vi "RegisterMap_Split RegMap.vi"(8 "error in (no error)":errorcluster, 11 "Register RegMap Strings":string[](array[string])) -> (0 "error out":errorcluster, 2 "Register RegMap Data":string[][](array[string]))   [LabVIEW 2010]
doc: "This VI splits the RegMap string from the text file into the individual bits/components.\n\nInputs:\nRegister RegMap Strings - (str[]) array of strings containing the specific register format for each of the regsiters in the register map file; rows = register and its format\nerror in - error input cluster\n\nOutputs:\nRegister RegMap Data - (str[]) 2-D array of strings with a element in the array for each register's format\nerror out - error output cluster"
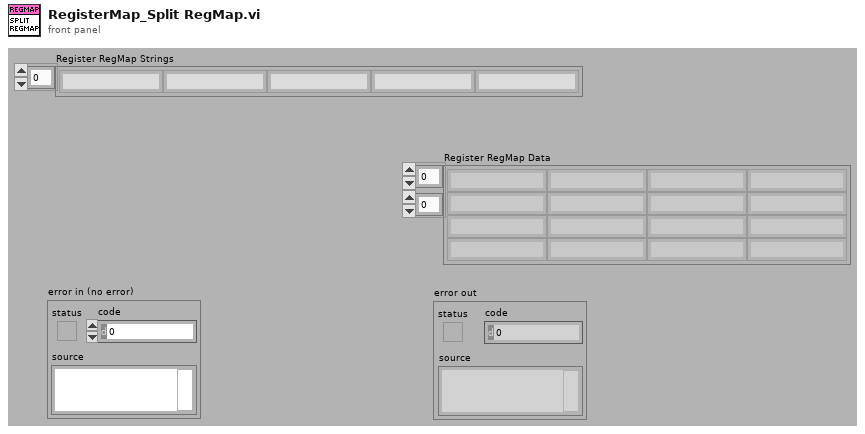
[diagram p1: front panel]
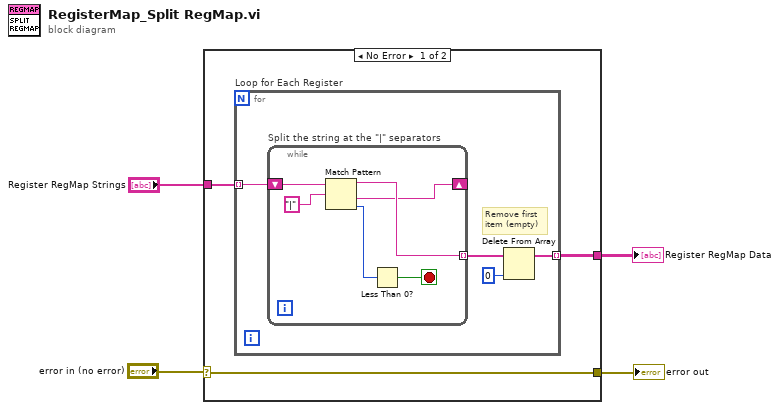
[diagram p0: block diagram]
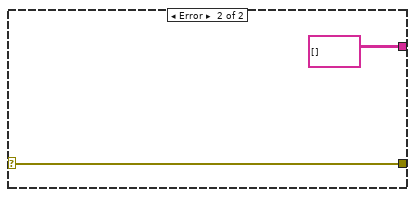
[diagram p2: hidden frame]
diagram:
  n1 = case shown="No Error" "error in (no error)" {
    selector: "error in (no error)" -> [w5 w19]
    tunnel: [w7 string[][] []] -> w4
    tunnel: "Register RegMap Strings" -> [w6 _]
    tunnel: [w5 w19] -> w1
    frame No Error {
      n2 = for "Loop for Each Register" {
        tunnel: w6 -> [w10] mode=indexing
        tunnel: [w11] -> w7 mode=indexing
        # "Remove first\nitem (empty)"
        n3 = while "Split the string at the \"|\" separators" {
          tunnel: [w14] -> w9 mode=indexing
          shift-right: [w12] -> _
          shift-left: w10 -> [w16]
          stop <- w17 stop-if-true
          n4 = Match Pattern(string=w16, regular expression="|" ("search string/char (-)")) -> (before substring=w14:string, after substring=w12:string, offset past match=w13:i32)  [unwired: 2 out]
          n5 = Less Than 0?(x=w13) -> (x < 0?=w17:bool)
        }
        n6 = Delete From Array(array=w9, index=0) -> (array with subset deleted=w11:string[])  [unwired: 1 in, 1 out]
      }
    }
    frame Error {
    }
  }
  "Register RegMap Data" <- w4
  "error out" <- w1
